vi "project!.vi"() -> ()   [LabVIEW 2014]
uses:
  <vilib>/picture/picture.llb/imagedata.ctl
  <vilib>/ptbypt/Frequency Domain.llb/Inverse Real FFT PtByPt.vi
  <vilib>/ptbypt/NI_PtbyPt.lvlib
panel:
  out "size(s) 3":i32[](array[numeric])
  out "Inverse FFT{X}":dbl[][](array[numeric])
  out "size(s) 2":i32
  out "Array":u8[](array[numeric])
  out "image":u8[](array[numeric])
  out "size(s)":i32
  out "image data":T1={"image type"=0, "image depth"=24, "image"=array[2359296 elements], "mask"=[], "colors"=[], "Rectangle"={"left"=0, "top"=0, "right"=1024, "bottom"=768}}
  in  "Path":path=path "U:/phys 434/Project/Desert.jpg"
  # "right=width\nbottom=height"
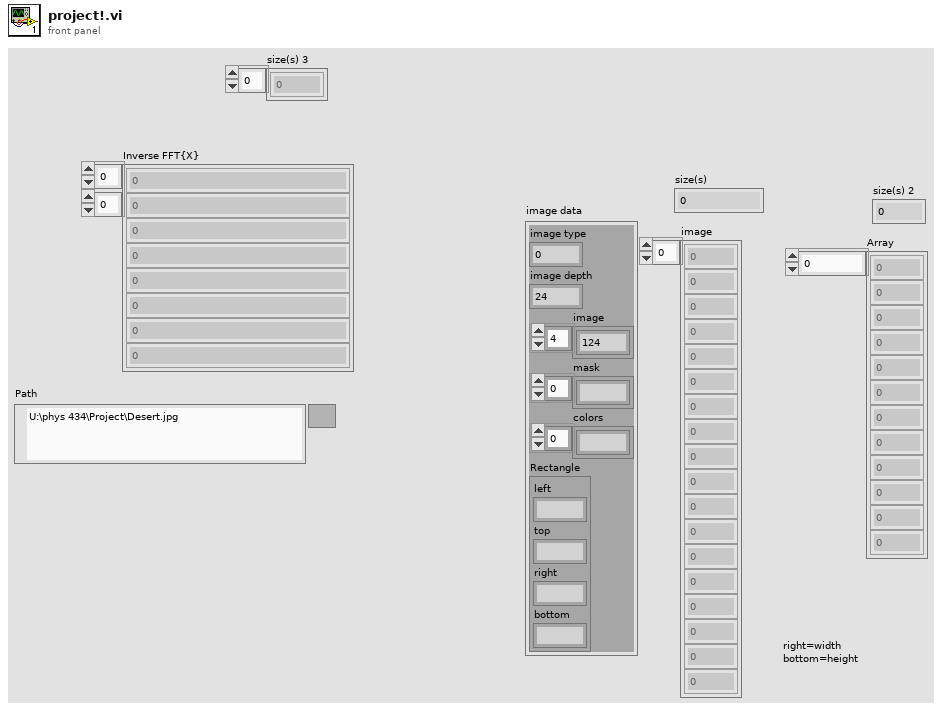
[diagram p1: front panel]
types:
  T1 = typedef "imagedata.ctl" = cluster{"image type":i32, "image depth":i32, "image":u8[], "mask":u8[], "colors":u32[], "Rectangle":cluster{"left":i16, "top":i16, "right":i16, "bottom":i16}}
  T2 = cluster{"left":i16, "top":i16, "right":i16, "bottom":i16}
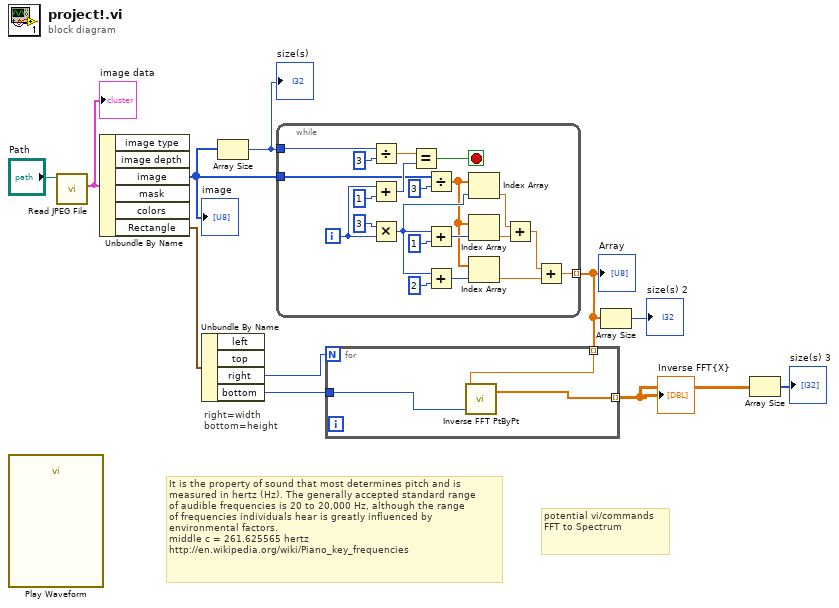
[diagram p0: block diagram]
diagram:
  # "right=width\nbottom=height"
  # "potential vi/commands\nFFT to Spectrum"
  # "It is the property of sound that most determines pitch and is \nmeasured in hertz (Hz). The generally accepted standard range \nof audible frequencies is 20 to 20,000 Hz, although the range \nof frequencies individuals hear is greatly influenced by \nenvironmental factors.\nmiddle c = 261.625565 hertz\nhttp://en.wikipedia.org/wiki/Piano_key_frequencies"
  n1 = call "Play Waveform"() -> ()  [unwired: 19 in, 1 out]
  n2 = call <vilib>:"Read JPEG File.vi"("path to JPEG file"="Path") -> ("image data"=w10:T1)  [unwired: 8 in, 2 out]
  "image data" <- w10
  n3 = Unbundle By Name(w10) -> ("image"=w8:u8[], "Rectangle"=w9:T2)  [unwired: 4 out]
  "image" <- w8
  n4 = Unbundle By Name(w9) -> ("right"=w4:i16, "bottom"=w5:i16)  [unwired: 2 out]
  n5 = Array Size(array=w8) -> (size(s)=w7:i32)
  "size(s)" <- w7
  n6 = while {
    tunnel: w8 -> [w15]
    tunnel: w7 -> [w22]
    tunnel: [w12] -> w3 mode=indexing
    i -> [w19]
    stop <- w20 stop-if-true
    n7 = Divide(x=w22, y=3) -> (x/y=w16:dbl)
    n8 = Add(x=w19, y=1) -> (x+y=w17:i32)
    n9 = Multiply(x=3, y=w19) -> (x*y=w27:i32)
    n10 = Equal?(x=w16, y=w17) -> (x = y?=w20:bool)
    n11 = Divide(x=w15, y=u8 3) -> (x/y=w13:dbl[])
    n12 = Add(x=w27, y=1) -> (x+y=w24:i32)
    n13 = Add(x=w27, y=2) -> (x+y=w23:i32)
    n14 = Index Array(array=w13, index=w27) -> (element=w32:dbl)
    n15 = Index Array(array=w13, index=w24) -> (element=w31:dbl)
    n16 = Index Array(array=w13, index=w23) -> (element=w30:dbl)
    n17 = Add(x=w32, y=w31) -> (x+y=w29:dbl)
    n18 = Add(x=w29, y=w30) -> (x+y=w12:dbl)
  }
  "Array" <- w3
  n19 = for {
    N: w4 -> [_]
    tunnel: w5 -> [w35]
    tunnel: w3 -> [w34] mode=indexing
    tunnel: [w33] -> w2 mode=indexing
    n20 = call-poly <vilib>:"Inverse FFT PtByPt.vi"("sample length"=w35, "x"=w34) -> ("Inverse FFT{X}"=w33:dbl[])  [unwired: 2 in, 1 out]
  }
  "Inverse FFT{X}" <- w2
  n21 = Array Size(array=w3) -> (size(s)=→"size(s) 2":i32)
  n22 = Array Size(array=w2) -> (size(s)=→"size(s) 3":i32[])
